vi "sever1.vi"() -> ()   [LabVIEW 2012]
panel:
  in  "读取的字节":i32
  out "数据输出":string
  in  "数据输入":string
  out "远程端口":u16
  out "远程地址":string
  in  "端口":u16
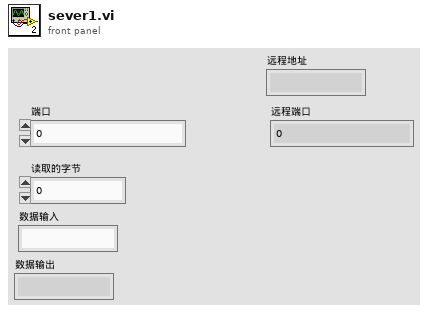
[diagram p1: front panel]
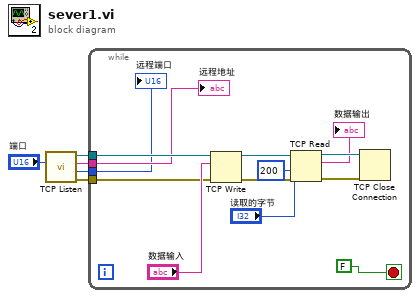
[diagram p0: block diagram]
diagram:
  n1 = call <vilib>:"TCP Listen.vi"("port"="端口") -> ("error out"=w3:errorcluster, "remote port"=w1:u16, "remote address"=w2:string, "connection ID"=w4:refnum<k5>)  [unwired: 6 in, 1 out]
  n2 = while {
    tunnel: w4 -> [w10]
    tunnel: w3 -> [w9]
    tunnel: w2 -> [w8]
    tunnel: w1 -> [w7]
    stop <- FALSE stop-if-true
    n3 = TCP Write(connection ID=w10, data in="数据输入", error in (no error)=w9) -> (connection ID out=w17:refnum<k5>, error out=w16:errorcluster)  [unwired: 1 in, 1 out]
    n4 = TCP Read(connection ID=w17, bytes to read="读取的字节", error in (no error)=w16, 9:200 ("超时毫秒(25000)")) -> (connection ID out=w15:refnum<k5>, data out=→"数据输出":string, error out=w14:errorcluster)  [unwired: 1 in]
    n5 = TCP Close Connection(connection ID=w15, error in (no error)=w14) -> ()  [unwired: 1 in, 2 out]
    "远程地址" <- w8
    "远程端口" <- w7
  }
